vi "Actor Core.vi"(8 "error in":errorcluster, 11 "Camera Settings Dialog in":refnum<class "Camera Settings Dialog.lvclass">) -> (0 "error out":errorcluster, 3 "Actor out":refnum<class "Actor.lvclass">)   [LabVIEW 2020, in "Camera Settings Dialog UI.lvlib" / "Camera Settings Dialog.lvclass"]
doc: "(<B>Filename</B>: Actor Framework.lvlib:Actor.lvclass:Actor Core.vi)\n\nReceives messages to the actor, reacts to them, and initiates any error handling that may shut the actor down.\n\nDescendant classes may override this VI to append parallel tasks for the actor to complete while it handles messages. Overrides use the Call Parent Method node."
uses:
  Camera Settings Dialog.lvclass
  <vilib>/ActorFramework/Actor/Actor.lvclass
  <vilib>/ActorFramework/Stop Msg/Stop Msg.lvclass
  Viewable Actor/ViewableActor/ViewableActor.lvclass
  Camera Settings Dialog Messages/Update Value Control Msg/Update Value Control Msg.lvclass
  Camera Settings Dialog Messages/Write Control Value to Cam Msg/Write Control Value to Cam Msg.lvclass
  Camera Settings Dialog Messages/Set Attr Filter Msg/Set Attr Filter Msg.lvclass
  C:/Users/AlexK/work/LabVIEW Programme/HIJ_Vision_Project_LV2020/Submodules/Viewable Actor/ViewableActor/ViewableActor.lvclass
  C:/Program Files (x86)/National Instruments/LabVIEW 2020/vi.lib/ActorFramework/Actor/Actor.lvclass
  C:/Users/AlexK/work/LabVIEW Programme/HIJ_Vision_Project_LV2020/Submodules/HIJ Vision/Camera Actors/Camera Settings Dialog UI/Camera Settings Dialog UI/Camera Settings Dialog.lvclass
panel:
  in  "Filter":string="exposure trigger"
  in  "Tab Control":T1(tab)
  in  "U32 Value Control":u32(slide) scale=4.0..4044.0
  in  "DBL Value Control":dbl(slide) min=17.00000029813964 max=5000000.0 step=1.0 scale=17.00000029813964..5000000.0
  in  "String Value Control":string
  in  "Enum Value Control":u32(ring) items=["Use hardware value", "10-bit", "12-bit", "14-bit", "16-bit"]
  in  "Boolean Value Control":bool=TRUE
  in  "Command Value Control":bool
  in  "Attribute Table":string(tree)="_1"
  out "Units":string
  out "Tooltip":string
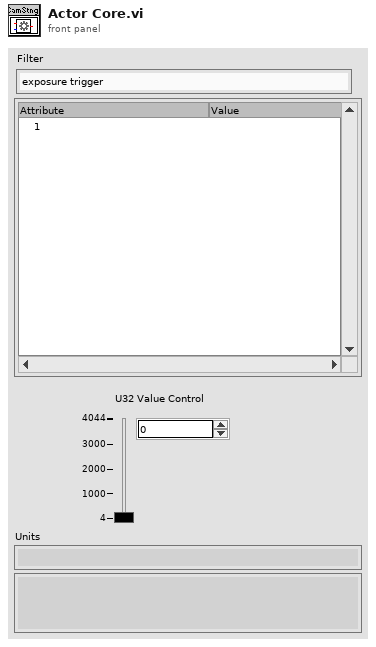
[diagram p1: front panel]
types:
  T1 = enum32{"U32", "DBL", "String", "Enum", "Bool", "Command"}
  T2 = cluster{"Tab Control":refnum<vi>, "U32 Value Control":refnum<vi>, "DBL Value Control":refnum<vi>, "String Value Control":refnum<vi>, "Enum Value Control":refnum<vi>, "Boolean Value Control":refnum<vi>, "Command Value Control":refnum<vi>}
  T3 = typedef "eventvkey.ctl" = enum16{"ASCII", "Enter", "Return", "Shift", "Ctrl", "Alt", "Cmd", "Opt", "Caps", "NumLock", "Clear", "Break", "Up", "Down", "Left", "Right", "Insert", "Delete", "Home", "End", "PageUp", "PageDown", "Escape", "Help", "Pause", "ScrollLock", "F1", "F2", "F3", "F4", "F5", "F6", "F7", "F8", "F9", "F10", "F11", "F12", "F13", "F14", "F15", "F16", "F17", "F18", "F19", "F20", "F21", "F22", "F23", "F24", "Play", "VolumeUp", "VolumeDown", "Mute", "Two Byte Char"}
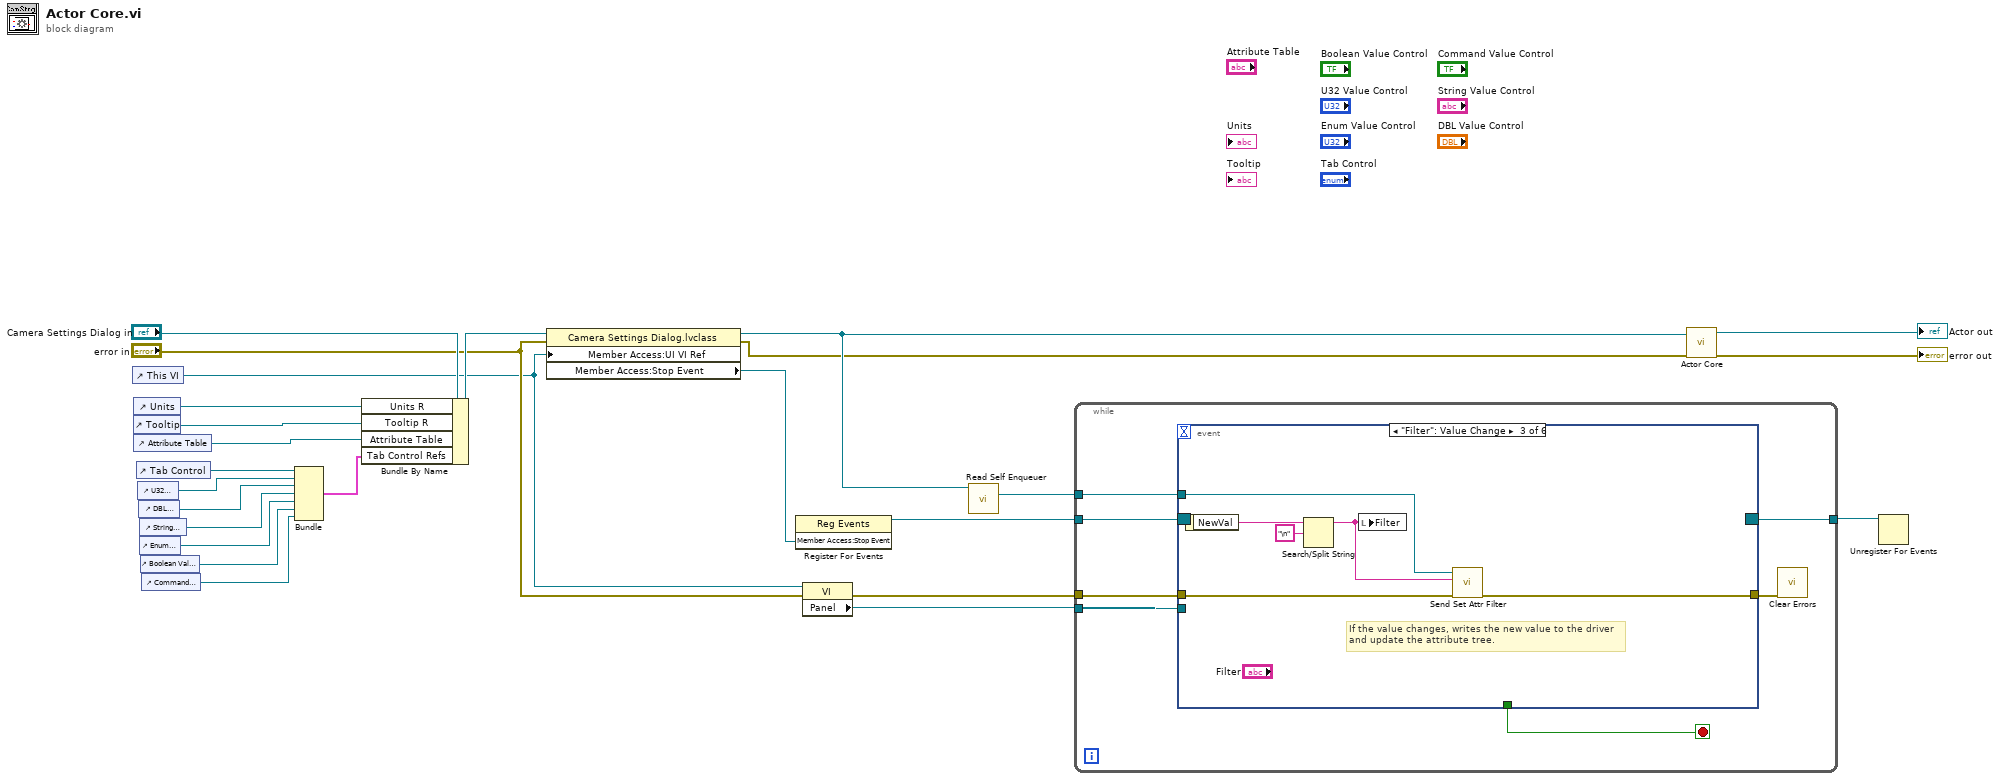
[diagram p0: block diagram]
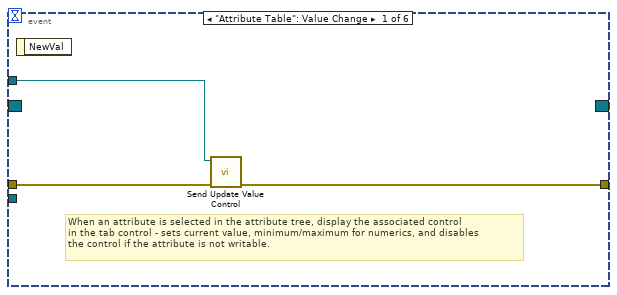
[diagram p2: hidden frame]
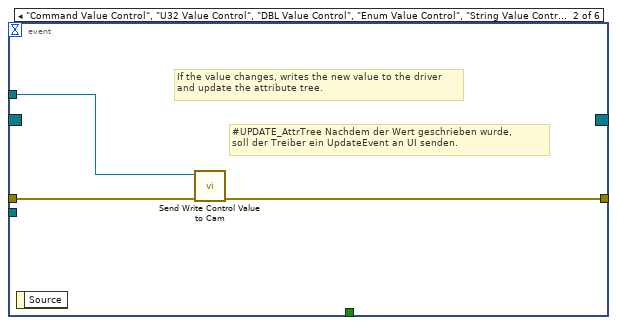
[diagram p3: hidden frame]
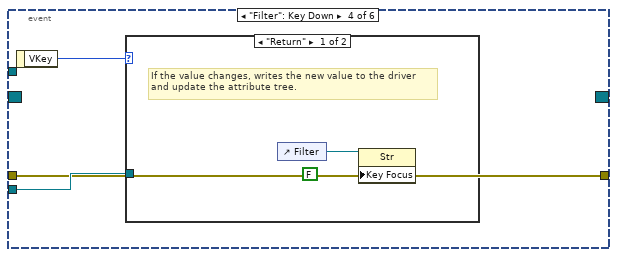
[diagram p4: hidden frame]
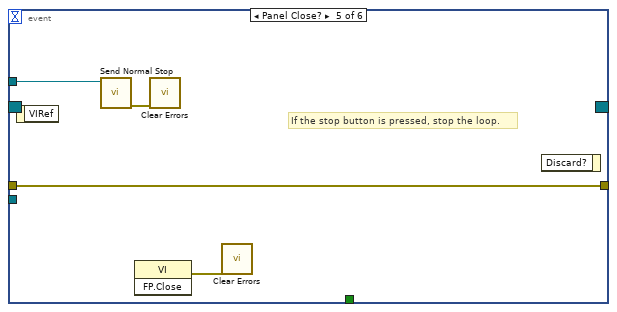
[diagram p6: hidden frame]
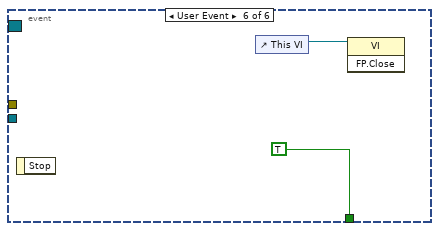
[diagram p7: hidden frame]
diagram:
  n1 = control-ref of="This VI"() -> (w5:refnum<vi>)
  n2 = control-ref of="Units"() -> (w2:refnum<vi>)
  n3 = control-ref of="Tooltip"() -> (w3:refnum<vi>)
  n4 = control-ref of="Attribute Table"() -> (w1:refnum<vi>)
  n5 = control-ref of="Tab Control"() -> (w13:refnum<vi>)
  n6 = control-ref of="U32 Value Control"() -> (w15:refnum<vi>)
  n7 = control-ref of="DBL Value Control"() -> (w16:refnum<vi>)
  n8 = control-ref of="String Value Control"() -> (w14:refnum<vi>)
  n9 = control-ref of="Enum Value Control"() -> (w17:refnum<vi>)
  n10 = control-ref of="Boolean Value Control"() -> (w18:refnum<vi>)
  n11 = control-ref of="Command Value Control"() -> (w19:refnum<vi>)
  n12 = Bundle("Tab Control"=w13, "U32 Value Control"=w15, "DBL Value Control"=w16, "String Value Control"=w14, "Enum Value Control"=w17, "Boolean Value Control"=w18, "Command Value Control"=w19) -> (w4:T2)  [unwired: 1 out]
  n13 = Bundle By Name(cluster="Camera Settings Dialog in", "Units R"=w2, "Tooltip R"=w3, "Attribute Table"=w1, "Tab Control Refs"=w4) -> (w25:refnum<class "Camera Settings Dialog.lvclass">)
  n14 = property class="Camera Settings Dialog.lvclass"(reference=w25, error in="error in", "Member Access:UI VI Ref"=w5) -> (reference out=w10:refnum<class "Camera Settings Dialog.lvclass">, error out=w9:errorcluster, "Member Access:Stop Event"=w8:refnum<user-event>)
  n15 = register-events(w8) -> (reference out=w7:refnum<event-registration>)  [unwired: 2 in, 1 out]
  n16 = property class="VI"(reference=w5, error in="error in") -> (error out=w21:errorcluster, "Panel"=w20:refnum<vi>)  [unwired: 1 out]
  n17 = call <vilib>:"Read Self Enqueuer.vi"("Actor"=w10) -> ("Self Enqueuer"=w11:refnum<class "Message Enqueuer.lvclass">)  [unwired: 10 in]
  n18 = while {
    tunnel: w21 -> [w32]
    tunnel: w20 -> [w31]
    tunnel: w11 -> [w28]
    tunnel: w7 -> [w27]
    tunnel: [w26] -> w6
    stop <- w30 stop-if-true
    n19 = event shown="[2] \"Filter\": Value Change" {
      selector: w27 -> [_ _ _ _ _ _]
      dyn-events: [_ _ _ _ _ _] -> w26
      timeout: _ -> [_ _ _ _ _ _]
      tunnel: w32 -> [w33 w38 w44 w46 w53 _]
      tunnel: [w34 w37 w41 w46 w53 _] -> w29
      tunnel: w31 -> [_ _ _ w47 _ _]
      tunnel: [_ _ _ _ _ TRUE ("stop")] -> w30
      tunnel: w28 -> [w35 w36 w40 _ w51 _]
      event "Attribute Table": Value Change {
        # "When an attribute is selected in the attribute tree, display the associated control\nin the tab control - sets current value, minimum/maximum for numerics, and disables\nthe control if the attribute is not writable."
        n20 = event-data() -> ()  [unwired: 2 out]
        n21 = call "Send Update Value Control.vi"("error in (no error)"=w33, "Message Enqueuer"=w35) -> ("error out"=w34:errorcluster)  [unwired: 8 in, 1 out]
      }
      event "Command Value Control", "U32 Value Control", "DBL Value Control", "Enum Value Control", "String Value Control": Value Change; "U32 Value Control", "DBL Value Control": Mouse Up {
        # "#UPDATE_AttrTree Nachdem der Wert geschrieben wurde,\nsoll der Treiber ein UpdateEvent an UI senden."
        # "If the value changes, writes the new value to the driver\nand update the attribute tree."
        n22 = event-data() -> ()  [unwired: 2 out]
        n23 = call "Send Write Control Value to Cam.vi"("error in (no error)"=w38, "Message Enqueuer"=w36) -> ("error out"=w37:errorcluster)  [unwired: 8 in, 1 out]
      }
      event "Filter": Value Change {
        # "If the value changes, writes the new value to the driver\nand update the attribute tree."
        n24 = event-data() -> ("NewVal"=w43:string)  [unwired: 1 out]
        n25 = Search/Split String(string=w43, search string/char (-)="\n") -> (substring before match=w39:string)  [unwired: 1 in, 2 out]
        n26 = local write "Filter"(w39) -> ()
        n27 = call "Send Set Attr Filter.vi"("error in (no error)"=w44, "Attr Filter"=w39, "Message Enqueuer"=w40) -> ("error out"=w41:errorcluster)  [unwired: 7 in, 1 out]
      }
      event "Filter": Key Down {
        n28 = event-data() -> ("VKey"=w45:T3)  [unwired: 1 out]
        n29 = case shown="\"Return\"" w45 {
          tunnel: w47 -> [_ _]
          frame "Return" {
            # "If the value changes, writes the new value to the driver\nand update the attribute tree."
            n30 = control-ref of="Filter"() -> (w48:refnum<vi>)
            n31 = property class="Str"(reference=w48, "Key Focus"=FALSE) -> ()  [unwired: 1 in, 2 out]
          }
          frame "Enter", Default {
          }
        }
      }
      event Panel Close? {
        # "If the stop button is pressed, stop the loop."
        n32 = event-data() -> ()  [unwired: 2 out]
        n33 = call <vilib>:"Send Normal Stop.vi"("Message Enqueuer"=w51) -> ("error out"=w50:errorcluster)  [unwired: 10 in]
        n34 = invoke class="VI" method="FP.Close"() -> (error out=w52:errorcluster)  [unwired: 3 in, 2 out]
        n35 = call <vilib>:"Clear Errors.vi"("error in (no error)"=w50) -> ()  [unwired: 5 in, 2 out]
        n36 = call <vilib>:"Clear Errors.vi"("error in (no error)"=w52) -> ()  [unwired: 5 in, 2 out]
        n37 = event-data() -> ()  [unwired: 2 in, 1 out]
      }
      event User Event {
        n38 = event-data() -> ()  [unwired: 2 out]
        n39 = control-ref of="This VI"() -> (w54:refnum<vi>)
        n40 = invoke class="VI" method="FP.Close"(reference=w54) -> ()  [unwired: 2 in, 3 out]
      }
    }
    n41 = call <vilib>:"Clear Errors.vi"("error in (no error)"=w29) -> ()  [unwired: 5 in, 2 out]
  }
  n42 = call-parent "Actor Core.vi"("error in"=w9, "Actor in"=w10) -> ("error out"=→"error out":errorcluster, "Actor out"=→"Actor out":refnum<class "Actor.lvclass">)  [unwired: 8 in]
  n43 = Unregister For Events(event registration refnum=w6) -> ()  [unwired: 1 in, 1 out]
